vi "H5Lget_val.vi"   [LabVIEW 2017]
doc: "Returns the value of a symbolic link."
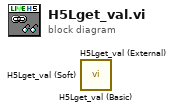
[diagram p0: block diagram]
diagram:
  n1 = call <vilib>:"H5Lget_val (Basic).vi"() -> ()  [unwired: 8 in, 4 out]
  n2 = call <vilib>:"H5Lget_val (External).vi"() -> ()  [unwired: 7 in, 5 out]
  n3 = call <vilib>:"H5Lget_val (Soft).vi"() -> ()  [unwired: 8 in, 4 out]
